vi "PXI-Prime DO.vi"(0 "DO Tasks":T1[](array[typedef]), 11 "error in":errorcluster) -> (4 "DO Tasks out":T1[](array[typedef]), 8 "DO Waveforms":bool[][](array[boolean]), 15 "error out":errorcluster)   [LabVIEW 2020]
uses:
  Type Defs/Task Struct.ctl
  Type Defs/PXI-DO Signal Bank Action.ctl
  PXI Globals.vi
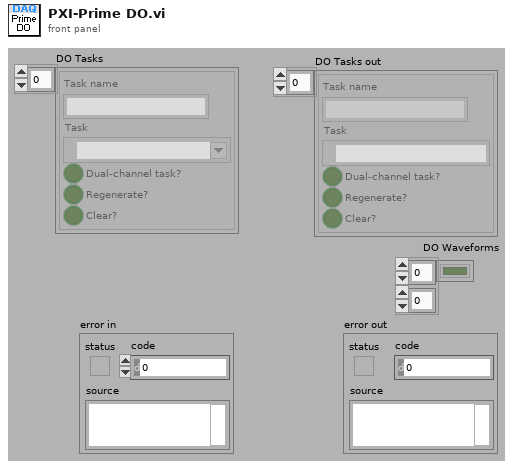
[diagram p1: front panel]
types:
  T1 = typedef "Task Struct.ctl" = cluster{"Task name":string, "Task":refnum<k21>, "Dual-channel task?":bool, "Regenerate?":bool, "Clear?":bool}
  T2 = typedef "PXI-DO Signal Bank Action.ctl" = enum16{"Clear", "Write", "Read"}
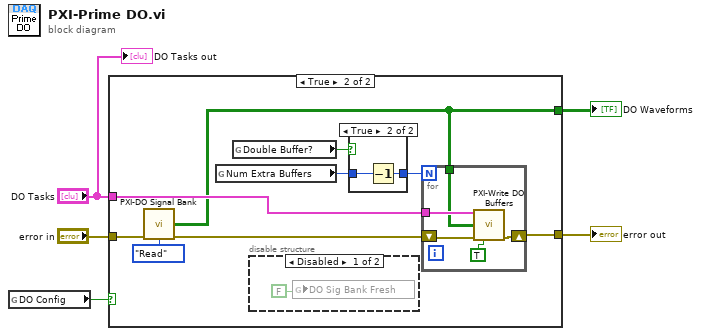
[diagram p0: block diagram]
diagram:
  n1 = global read "PXI Globals.vi" "DO Config"() -> (w5:bool)
  n2 = case shown="True" w5 {
    tunnel: "error in" -> [w6 w10]
    tunnel: [w6 w15] -> w4
    tunnel: "DO Tasks" -> [_ w11]
    tunnel: [_ w7] -> w1
    frame False {
    }
    frame True {
      n3 = call "PXI-DO Signal Bank.vi"("error in (no error)"=w10, "Action"=PXI-DO_Signal_Bank_Action."Read") -> ("Array out"=w7:bool[][], "error out"=w8:errorcluster)  [unwired: 12 in]
      n4 = global read "PXI Globals.vi" "Num Extra Buffers"() -> (w12:i32)
      n5 = global read "PXI Globals.vi" "Double Buffer?"() -> (w13:bool)
      n6 = disable-structure shown="Disabled" {
        frame Disabled {
          n7 = global write "PXI Globals.vi" "DO Sig Bank Fresh"(FALSE) -> ()
        }
        frame Enabled {
        }
      }
      n8 = case shown="True" w13 {
        tunnel: [w17 w19] -> w14
        tunnel: w12 -> [w17 w18]
        frame False {
        }
        frame True {
          n9 = Decrement(x=w18) -> (x-1=w19:i32)
        }
      }
      n10 = for {
        N: w14 -> [_]
        shift-right: [w24] -> w15
        shift-left: w8 -> [w23]
        tunnel: w7 -> [w20]
        tunnel: w11 -> [w22]
        n11 = call "PXI-Write DO Buffers.vi"("DO Tasks"=w22, "DO Waveforms"=w20, "error in (no error)"=w23, "Force write"=TRUE) -> ("error out"=w24:errorcluster)  [unwired: 10 in, 1 out]
      }
    }
  }
  "error out" <- w4
  "DO Waveforms" <- w1
  "DO Tasks out" <- "DO Tasks"
